vi "ClusterToContent.vi"(11 "Cluster":T1) -> (3 "Content":string)   [LabVIEW 2020]
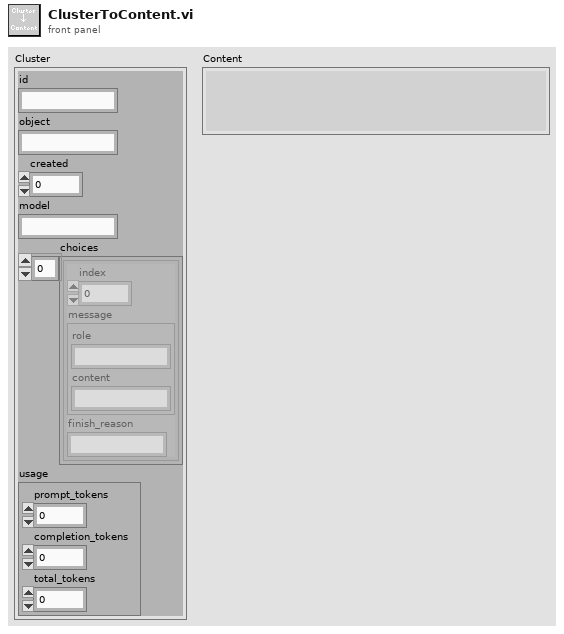
[diagram p1: front panel]
types:
  T1 = cluster{"id":string, "object":string, "created":i32, "model":string, "choices":cluster{"index":i32, "message":cluster{"role":string, "content":string}, "finish_reason":string}[], "usage":cluster{"prompt_tokens":i32, "completion_tokens":i32, "total_tokens":i32}}
  T2 = cluster{"index":i32, "message":cluster{"role":string, "content":string}, "finish_reason":string}[]
  T3 = cluster{"index":i32, "message":cluster{"role":string, "content":string}, "finish_reason":string}
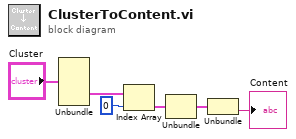
[diagram p0: block diagram]
diagram:
  n1 = Unbundle("Cluster") -> ("choices"=w2:T2)  [unwired: 5 out]
  n2 = Index Array(array=w2, index=0) -> (element=w4:T3)
  n3 = Unbundle(w4) -> ("message"=w5:cluster{"role":string, "content":string})  [unwired: 2 out]
  n4 = Unbundle(w5) -> ("content"=→"Content":string)  [unwired: 1 out]
